vi "Markowski Smoothing.vi"(7 "smooth":u8, 10 "IV in":sgl[](array[numeric]), 11 "DMA in":refnum<class "DMA.lvclass">) -> (1 "Finished?":bool, 2 "IV Out":sgl[](array[numeric]), 3 "DMA Out":refnum<class "DMA.lvclass">)   [LabVIEW 2015, in "DMA.lvclass"]
uses:
  DMA.lvclass
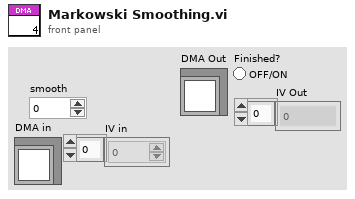
[diagram p1: front panel]
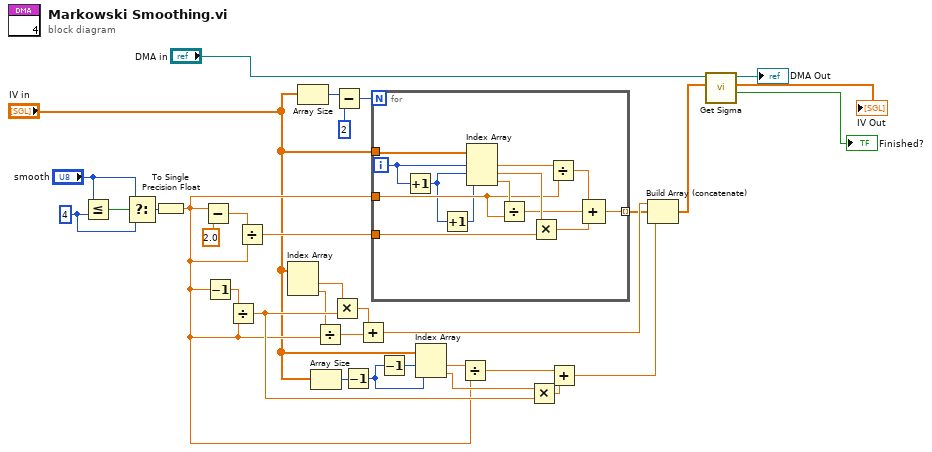
[diagram p0: block diagram]
diagram:
  w8 = u8 4 ("y")
  n1 = Less Or Equal?(x="smooth", y=w8) -> (x <= y?=w6:bool)
  n2 = Select(t="smooth", s=w6, f=w8) -> (s? t:f=w9:u8)
  n3 = To Single Precision Float(number=w9) -> (single precision float=w27:sgl)
  n4 = Subtract(x=w27, y=sgl 2.0) -> (x-y=w11:sgl)
  n5 = Decrement(x=w27) -> (x-1=w16:sgl)
  n6 = Divide(x=w16, y=w27) -> (x/y=w29:sgl)
  n7 = Divide(x=w11, y=w27) -> (x/y=w15:sgl)
  n8 = Index Array(array="IV in") -> (element #1=w17:sgl, element #2=w18:sgl)  [unwired: 2 in]
  n9 = Array Size(array="IV in") -> (size(s)=w12:i32)
  n10 = Array Size(array="IV in") -> (size(s)=w23:i32)
  n11 = Divide(x=w18, y=w27) -> (x/y=w21:sgl)
  n12 = Multiply(x=w17, y=w29) -> (x*y=w20:sgl)
  n13 = Subtract(x=w12, y=2) -> (x-y=w14:i32)
  n14 = Decrement(x=w23) -> (x-1=w25:i32)
  n15 = Add(x=w20, y=w21) -> (x+y=w22:sgl)
  n16 = for {
    N: w14 -> [_]
    tunnel: "IV in" -> [w46]
    tunnel: w27 -> [w41]
    tunnel: w15 -> [w43]
    tunnel: [w37] -> w19 mode=indexing
    i -> [w36]
    n17 = Increment(x=w36) -> (x+1=w35:i32)
    n18 = Increment(x=w35) -> (x+1=w34:i32)
    n19 = Index Array(array=w46, index #1=w36, index #2=w35, index #3=w34) -> (element #1=w45:sgl, element #2=w44:sgl, element #3=w42:sgl)
    n20 = Divide(x=w42, y=w41) -> (x/y=w39:sgl)
    n21 = Multiply(x=w44, y=w43) -> (x*y=w38:sgl)
    n22 = Divide(x=w45, y=w41) -> (x/y=w40:sgl)
    n23 = Compound Arithmetic op=ADD(w40, w39, w38) -> (w37:sgl)
  }
  n24 = Decrement(x=w25) -> (x-1=w24:i32)
  n25 = Index Array(array="IV in", index #1=w24, index #2=w25) -> (element #1=w26:sgl, element #2=w28:sgl)
  n26 = Divide(x=w26, y=w27) -> (x/y=w31:sgl)
  n27 = Multiply(x=w28, y=w29) -> (x*y=w30:sgl)
  n28 = Add(x=w31, y=w30) -> (x+y=w32:sgl)
  n29 = Build Array (concatenate)(w22, w19, w32) -> (w33:sgl[])
  n30 = call "Get Sigma.vi"("IV in"=w33, "DMA in"="DMA in") -> ("Finished?"=→"Finished?":bool, "IV Out"=→"IV Out":sgl[], "DMA Out"=→"DMA Out":refnum<class "DMA.lvclass">)  [unwired: 6 in, 1 out]
